vi "Error Write Status.vi"(8 "error in":errorcluster, 10 "Error STS":i32[](array[numeric]), 11 "Power Supply In":refnum<class "Power Supply.lvclass">) -> (0 "error out":errorcluster, 3 "Power Supply Out":refnum<class "Power Supply.lvclass">)   [LabVIEW 2023, in "Power Supply.lvclass"]
uses:
  Power Supply.lvclass
  Power Supply.lvclass/Power Supply.ctl
  Low Level Capabilities/Error/Error.lvclass
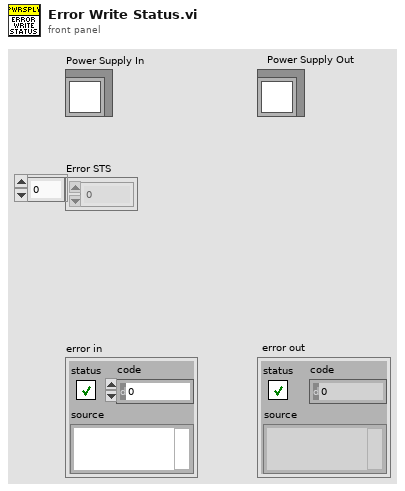
[diagram p1: front panel]
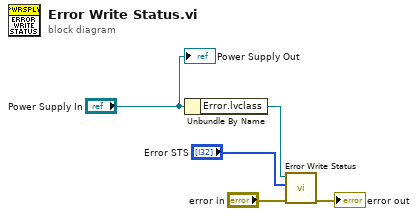
[diagram p0: block diagram]
diagram:
  n1 = Unbundle By Name("Power Supply In") -> ("Error.lvclass"=w4:refnum<class "Error.lvclass">)
  n2 = call-dynamic "Error Write Status.vi"("error in"="error in", "Error STS"="Error STS", "Error in"=w4) -> ("error out"=→"error out":errorcluster)  [unwired: 7 in, 1 out]
  "Power Supply Out" <- "Power Supply In"
